vi "ELVIS III v1.0 Build MUX Configuration Encoder.vi"(11 "Channel":T4) -> (1 "Configuration Bitmask Array":bool[][](array[boolean]), 2 "Configuration BitCode Array":bool[][](array[boolean]), 3 "Channel Reservation List":T1)   [LabVIEW 2021]
uses:
  <vilib>/myRIO/Common/Instrument Driver Framework/myRIO v1.0/Encoder/typedefs/Encoder Channels Enum.ctl
  <vilib>/myRIO/Common/Instrument Driver Framework/ELVIS III v1.0/Resource Manager/typedefs/ELVIS III v1.0 Channel Reservation List.ctl
  <vilib>/myRIO/Common/Instrument Driver Framework/ELVIS III v1.0/Resource Manager/typedefs/ELVIS III v1.0 Channel Reservation Info.ctl
  <vilib>/myRIO/Common/Instrument Driver Framework/ELVIS III v1.0/Resource Manager/typedefs/ELVIS III v1.0 Connector List.ctl
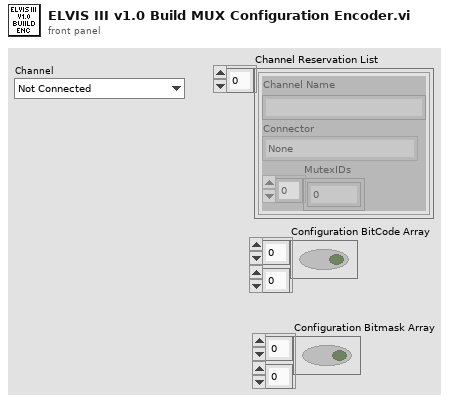
[diagram p1: front panel]
types:
  T1 = typedef "ELVIS III v1.0 Channel Reservation List.ctl" = T2[]
  T2 = typedef "ELVIS III v1.0 Channel Reservation Info.ctl" = cluster{"Channel Name":string, "Connector":T3, "MutexIDs":u32[]}
  T3 = typedef "ELVIS III v1.0 Connector List.ctl" = enum32{"None", "ConnectorA", "ConnectorB"}
  T4 = typedef "Encoder Channels Enum.ctl" = enum16{"Not Connected", "C/ENC0", "C/ENC1", "A/ENC", "A/ENC0", "A/ENC1", "A/ENC2", "A/ENC3", "A/ENC4", "A/ENC5", "A/ENC6", "A/ENC7", "A/ENC8", "A/ENC9", "B/ENC", "B/ENC0", "B/ENC1", "B/ENC2", "B/ENC3", "B/ENC4", "B/ENC5", "B/ENC6", "B/ENC7", "B/ENC8", "B/ENC9", "DIO/ENC0", "DIO/ENC1", "DIO/ENC2", "DIO/ENC3", "DIO/ENC4"}
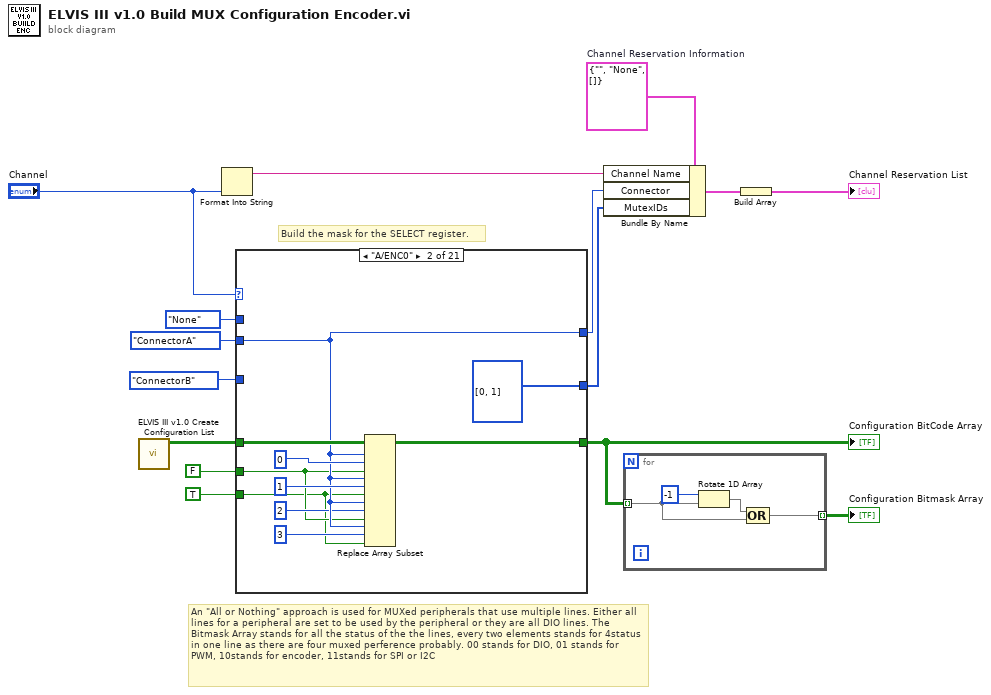
[diagram p0: block diagram]
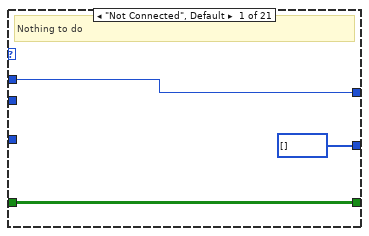
[diagram p2: hidden frame]
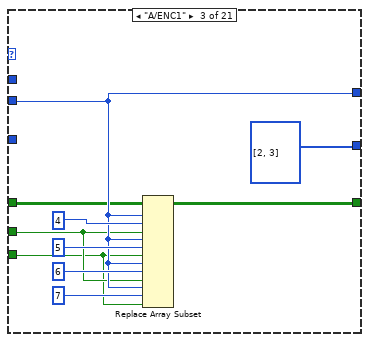
[diagram p3: hidden frame]
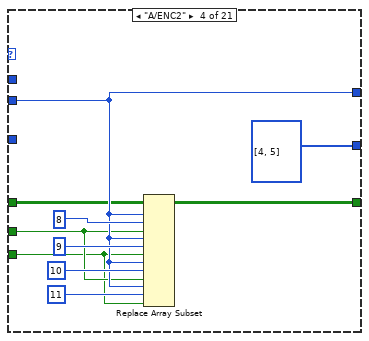
[diagram p4: hidden frame]
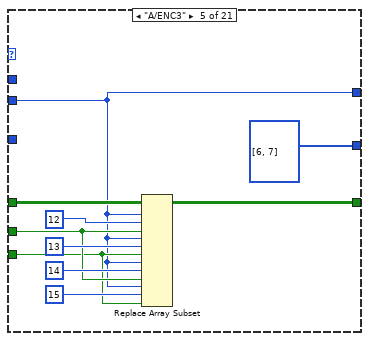
[diagram p5: hidden frame]
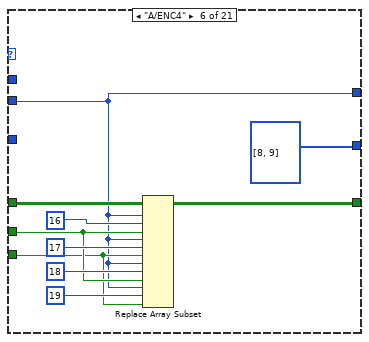
[diagram p6: hidden frame]
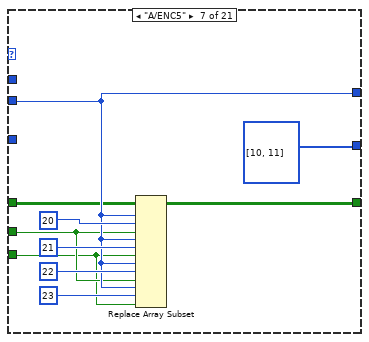
[diagram p7: hidden frame]
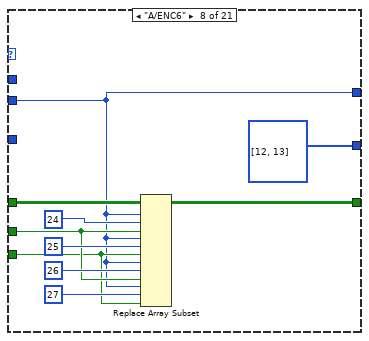
[diagram p8: hidden frame]
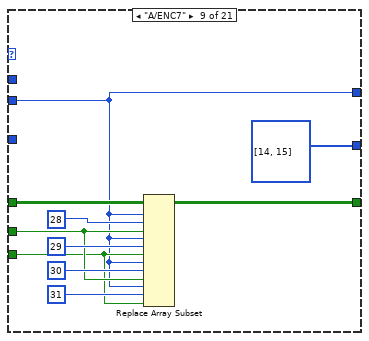
[diagram p9: hidden frame]
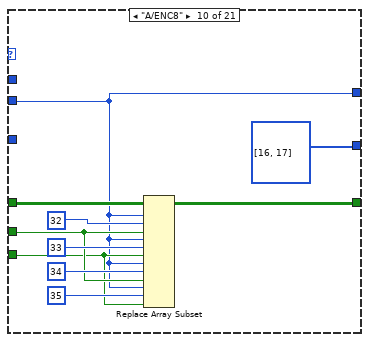
[diagram p10: hidden frame]
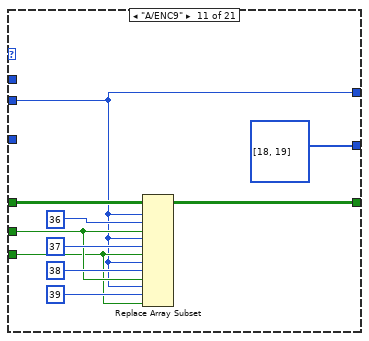
[diagram p11: hidden frame]
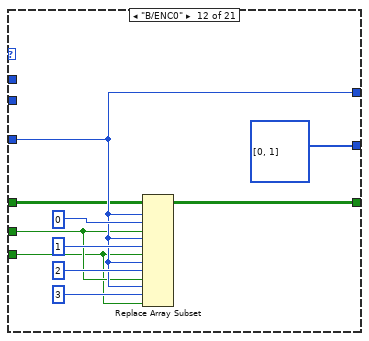
[diagram p12: hidden frame]
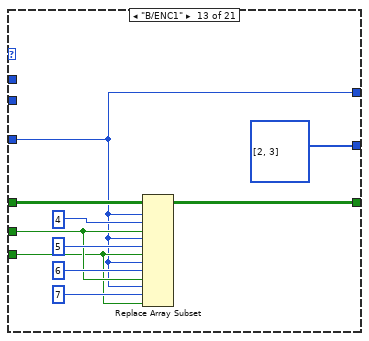
[diagram p13: hidden frame]
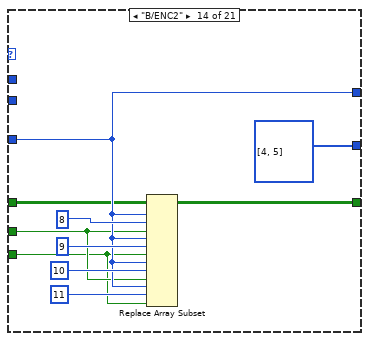
[diagram p14: hidden frame]
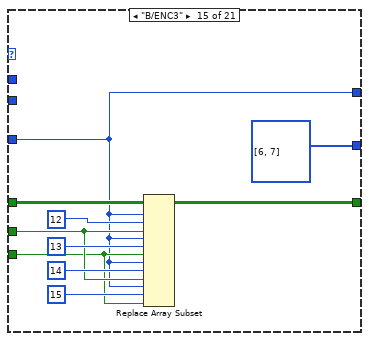
[diagram p15: hidden frame]
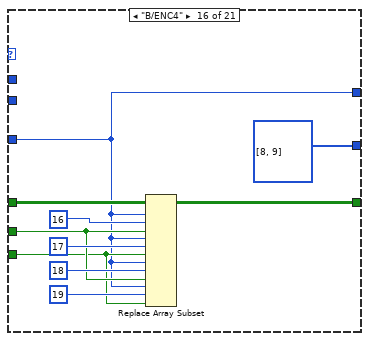
[diagram p16: hidden frame]
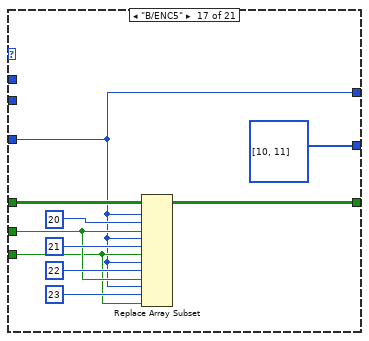
[diagram p17: hidden frame]
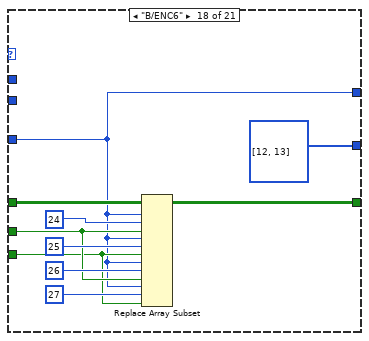
[diagram p18: hidden frame]
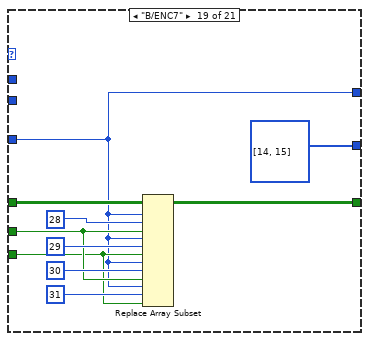
[diagram p19: hidden frame]
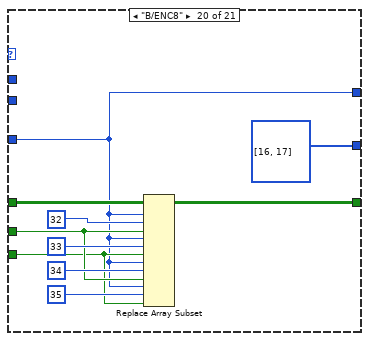
[diagram p20: hidden frame]
diagram:
  w7 = T2 {"Channel Name"="", "Connector"=enum."None", "MutexIDs"=[]}  # Channel Reservation Information
  # "An \"All or Nothing\" approach is used for MUXed peripherals that use multiple lines. Either all lines for a peripheral are set to be used by the peripheral or they are all DIO lines. The Bitmask Array stands for all the status of the the lines, every two elements stands for 4status in one line as there are four muxed perference probably. 00 stands for DIO, 01 stands for PWM, 10stands for encoder, 11stands for SPI or I2C"
  # "Build the mask for the SELECT register."
  n1 = call <vilib>:"ELVIS III v1.0 Create Configuration List.vi"() -> ("Bitmask Array"=w8:bool[][])  [unwired: 11 in]
  n2 = Format Into String("Channel") -> (resulting string=w12:string)  [unwired: 3 in, 1 out]
  n3 = case shown="\"A/ENC0\"" "Channel" {
    tunnel: w8 -> [w18 w24 w31 w41 w54 w64 w71 w84 w94 w104 w114 w121 w134 w141 w154 w164 w174 w184 w194 w204 w214]
    tunnel: [w18 w25 w32 w42 w51 w61 w72 w79 w89 w101 w111 w122 w131 w142 w151 w161 w171 w181 w189 w201 w211] -> w2
    tunnel: ELVIS_III_v1.0_Connector_List."None" ("Connector List") -> [w17 _ _ _ _ _ _ _ _ _ _ _ _ _ _ _ _ _ _ _ _]
    tunnel: ELVIS_III_v1.0_Connector_List."ConnectorA" ("Connector List") -> [_ w23 w34 w44 w50 w59 w74 w81 w90 w100 w109 _ _ _ _ _ _ _ _ _ _]
    tunnel: TRUE ("new element/subarray") -> [_ w19 w29 w39 w52 w62 w69 w82 w92 w102 w112 w119 w132 w139 w152 w162 w172 w182 w192 w202 w212]
    tunnel: [w17 w23 w34 w44 w50 w59 w74 w81 w90 w100 w109 w124 w129 w144 w149 w159 w169 w179 w191 w199 w209] -> w9
    tunnel: ELVIS_III_v1.0_Connector_List."ConnectorB" ("Connector List") -> [_ _ _ _ _ _ _ _ _ _ _ w124 w129 w144 w149 w159 w169 w179 w191 w199 w209]
    tunnel: [u32[] [] u32[] [0, 1] u32[] [2, 3] u32[] [4, 5] u32[] [6, 7] u32[] [8, 9] u32[] [10, 11] u32[] [12, 13] u32[] [14, 15] u32[] [16, 17] u32[] [18, 19] u32[] [0, 1] u32[] [2, 3] u32[] [4, 5] u32[] [6, 7] u32[] [8, 9] u32[] [10, 11] u32[] [12, 13] u32[] [14, 15] u32[] [16, 17] u32[] [18, 19]] -> w4
    tunnel: FALSE ("new element/subarray") -> [_ w20 w30 w40 w53 w63 w70 w83 w93 w103 w113 w120 w133 w140 w153 w163 w173 w183 w193 w203 w213]
    frame "Not Connected", Default {
      # "Nothing to do"
    }
    frame "A/ENC0" {
      n4 = Replace Array Subset(array=w24, new element #1=w20, index (row) #1=w23, index (col) #1=0 ("disabled index (col)"), new element #2=w19, index (row) #2=w23, index (col) #2=1 ("disabled index (col)"), new element #3=w20, index (row) #3=w23, index (col) #3=2 ("disabled index (col)"), new element #4=w19, index (row) #4=w23, index (col) #4=3 ("disabled index (col)")) -> (w25:bool[][])
    }
    frame "A/ENC1" {
      n5 = Replace Array Subset(array=w31, new element #1=w30, index (row) #1=w34, index (col) #1=4 ("disabled index (col)"), new element #2=w29, index (row) #2=w34, index (col) #2=5 ("disabled index (col)"), new element #3=w30, index (row) #3=w34, index (col) #3=6 ("disabled index (col)"), new element #4=w29, index (row) #4=w34, index (col) #4=7 ("disabled index (col)")) -> (w32:bool[][])
    }
    frame "A/ENC2" {
      n6 = Replace Array Subset(array=w41, new element #1=w40, index (row) #1=w44, index (col) #1=8 ("disabled index (col)"), new element #2=w39, index (row) #2=w44, index (col) #2=9 ("disabled index (col)"), new element #3=w40, index (row) #3=w44, index (col) #3=10 ("disabled index (col)"), new element #4=w39, index (row) #4=w44, index (col) #4=11 ("disabled index (col)")) -> (w42:bool[][])
    }
    frame "A/ENC3" {
      n7 = Replace Array Subset(array=w54, new element #1=w53, index (row) #1=w50, index (col) #1=12 ("disabled index (col)"), new element #2=w52, index (row) #2=w50, index (col) #2=13 ("disabled index (col)"), new element #3=w53, index (row) #3=w50, index (col) #3=14 ("disabled index (col)"), new element #4=w52, index (row) #4=w50, index (col) #4=15 ("disabled index (col)")) -> (w51:bool[][])
    }
    frame "A/ENC4" {
      n8 = Replace Array Subset(array=w64, new element #1=w63, index (row) #1=w59, index (col) #1=16 ("disabled index (col)"), new element #2=w62, index (row) #2=w59, index (col) #2=17 ("disabled index (col)"), new element #3=w63, index (row) #3=w59, index (col) #3=18 ("disabled index (col)"), new element #4=w62, index (row) #4=w59, index (col) #4=19 ("disabled index (col)")) -> (w61:bool[][])
    }
    frame "A/ENC5" {
      n9 = Replace Array Subset(array=w71, new element #1=w70, index (row) #1=w74, index (col) #1=20 ("disabled index (col)"), new element #2=w69, index (row) #2=w74, index (col) #2=21 ("disabled index (col)"), new element #3=w70, index (row) #3=w74, index (col) #3=22 ("disabled index (col)"), new element #4=w69, index (row) #4=w74, index (col) #4=23 ("disabled index (col)")) -> (w72:bool[][])
    }
    frame "A/ENC6" {
      n10 = Replace Array Subset(array=w84, new element #1=w83, index (row) #1=w81, index (col) #1=24 ("disabled index (col)"), new element #2=w82, index (row) #2=w81, index (col) #2=25 ("disabled index (col)"), new element #3=w83, index (row) #3=w81, index (col) #3=26 ("disabled index (col)"), new element #4=w82, index (row) #4=w81, index (col) #4=27 ("disabled index (col)")) -> (w79:bool[][])
    }
    frame "A/ENC7" {
      n11 = Replace Array Subset(array=w94, new element #1=w93, index (row) #1=w90, index (col) #1=28 ("disabled index (col)"), new element #2=w92, index (row) #2=w90, index (col) #2=29 ("disabled index (col)"), new element #3=w93, index (row) #3=w90, index (col) #3=30 ("disabled index (col)"), new element #4=w92, index (row) #4=w90, index (col) #4=31 ("disabled index (col)")) -> (w89:bool[][])
    }
    frame "A/ENC8" {
      n12 = Replace Array Subset(array=w104, new element #1=w103, index (row) #1=w100, index (col) #1=32 ("disabled index (col)"), new element #2=w102, index (row) #2=w100, index (col) #2=33 ("disabled index (col)"), new element #3=w103, index (row) #3=w100, index (col) #3=34 ("disabled index (col)"), new element #4=w102, index (row) #4=w100, index (col) #4=35 ("disabled index (col)")) -> (w101:bool[][])
    }
    frame "A/ENC9" {
      n13 = Replace Array Subset(array=w114, new element #1=w113, index (row) #1=w109, index (col) #1=36 ("disabled index (col)"), new element #2=w112, index (row) #2=w109, index (col) #2=37 ("disabled index (col)"), new element #3=w113, index (row) #3=w109, index (col) #3=38 ("disabled index (col)"), new element #4=w112, index (row) #4=w109, index (col) #4=39 ("disabled index (col)")) -> (w111:bool[][])
    }
    frame "B/ENC0" {
      n14 = Replace Array Subset(array=w121, new element #1=w120, index (row) #1=w124, index (col) #1=0 ("disabled index (col)"), new element #2=w119, index (row) #2=w124, index (col) #2=1 ("disabled index (col)"), new element #3=w120, index (row) #3=w124, index (col) #3=2 ("disabled index (col)"), new element #4=w119, index (row) #4=w124, index (col) #4=3 ("disabled index (col)")) -> (w122:bool[][])
    }
    frame "B/ENC1" {
      n15 = Replace Array Subset(array=w134, new element #1=w133, index (row) #1=w129, index (col) #1=4 ("disabled index (col)"), new element #2=w132, index (row) #2=w129, index (col) #2=5 ("disabled index (col)"), new element #3=w133, index (row) #3=w129, index (col) #3=6 ("disabled index (col)"), new element #4=w132, index (row) #4=w129, index (col) #4=7 ("disabled index (col)")) -> (w131:bool[][])
    }
    frame "B/ENC2" {
      n16 = Replace Array Subset(array=w141, new element #1=w140, index (row) #1=w144, index (col) #1=8 ("disabled index (col)"), new element #2=w139, index (row) #2=w144, index (col) #2=9 ("disabled index (col)"), new element #3=w140, index (row) #3=w144, index (col) #3=10 ("disabled index (col)"), new element #4=w139, index (row) #4=w144, index (col) #4=11 ("disabled index (col)")) -> (w142:bool[][])
    }
    frame "B/ENC3" {
      n17 = Replace Array Subset(array=w154, new element #1=w153, index (row) #1=w149, index (col) #1=12 ("disabled index (col)"), new element #2=w152, index (row) #2=w149, index (col) #2=13 ("disabled index (col)"), new element #3=w153, index (row) #3=w149, index (col) #3=14 ("disabled index (col)"), new element #4=w152, index (row) #4=w149, index (col) #4=15 ("disabled index (col)")) -> (w151:bool[][])
    }
    frame "B/ENC4" {
      n18 = Replace Array Subset(array=w164, new element #1=w163, index (row) #1=w159, index (col) #1=16 ("disabled index (col)"), new element #2=w162, index (row) #2=w159, index (col) #2=17 ("disabled index (col)"), new element #3=w163, index (row) #3=w159, index (col) #3=18 ("disabled index (col)"), new element #4=w162, index (row) #4=w159, index (col) #4=19 ("disabled index (col)")) -> (w161:bool[][])
    }
    frame "B/ENC5" {
      n19 = Replace Array Subset(array=w174, new element #1=w173, index (row) #1=w169, index (col) #1=20 ("disabled index (col)"), new element #2=w172, index (row) #2=w169, index (col) #2=21 ("disabled index (col)"), new element #3=w173, index (row) #3=w169, index (col) #3=22 ("disabled index (col)"), new element #4=w172, index (row) #4=w169, index (col) #4=23 ("disabled index (col)")) -> (w171:bool[][])
    }
    frame "B/ENC6" {
      n20 = Replace Array Subset(array=w184, new element #1=w183, index (row) #1=w179, index (col) #1=24 ("disabled index (col)"), new element #2=w182, index (row) #2=w179, index (col) #2=25 ("disabled index (col)"), new element #3=w183, index (row) #3=w179, index (col) #3=26 ("disabled index (col)"), new element #4=w182, index (row) #4=w179, index (col) #4=27 ("disabled index (col)")) -> (w181:bool[][])
    }
    frame "B/ENC7" {
      n21 = Replace Array Subset(array=w194, new element #1=w193, index (row) #1=w191, index (col) #1=28 ("disabled index (col)"), new element #2=w192, index (row) #2=w191, index (col) #2=29 ("disabled index (col)"), new element #3=w193, index (row) #3=w191, index (col) #3=30 ("disabled index (col)"), new element #4=w192, index (row) #4=w191, index (col) #4=31 ("disabled index (col)")) -> (w189:bool[][])
    }
    frame "B/ENC8" {
      n22 = Replace Array Subset(array=w204, new element #1=w203, index (row) #1=w199, index (col) #1=32 ("disabled index (col)"), new element #2=w202, index (row) #2=w199, index (col) #2=33 ("disabled index (col)"), new element #3=w203, index (row) #3=w199, index (col) #3=34 ("disabled index (col)"), new element #4=w202, index (row) #4=w199, index (col) #4=35 ("disabled index (col)")) -> (w201:bool[][])
    }
    frame "B/ENC9" {
      n23 = Replace Array Subset(array=w214, new element #1=w213, index (row) #1=w209, index (col) #1=36 ("disabled index (col)"), new element #2=w212, index (row) #2=w209, index (col) #2=37 ("disabled index (col)"), new element #3=w213, index (row) #3=w209, index (col) #3=38 ("disabled index (col)"), new element #4=w212, index (row) #4=w209, index (col) #4=39 ("disabled index (col)")) -> (w211:bool[][])
    }
  }
  "Configuration BitCode Array" <- w2
  n24 = Bundle By Name(cluster=w7, "Channel Name"=w12, "Connector"=w9, "MutexIDs"=w4) -> (w11:T2)
  n25 = for {
    tunnel: w2 -> [w220] mode=indexing
    tunnel: [w219] -> w1 mode=indexing
    n26 = Rotate 1D Array(1:w220, 2:-1 ("n")) -> (0:w221:bool[])
    n27 = Compound Arithmetic op=OR(w221, w220) -> (w219:bool[])
  }
  "Configuration Bitmask Array" <- w1
  n28 = Build Array(w11) -> (→"Channel Reservation List":T2[])
